vi "recommenceAt.vi"(7 "splitAtFile":path, 10 "Array":path[](array[path])) -> (2 "Array 2":path[](array[path]))   [LabVIEW 2022 SP3]
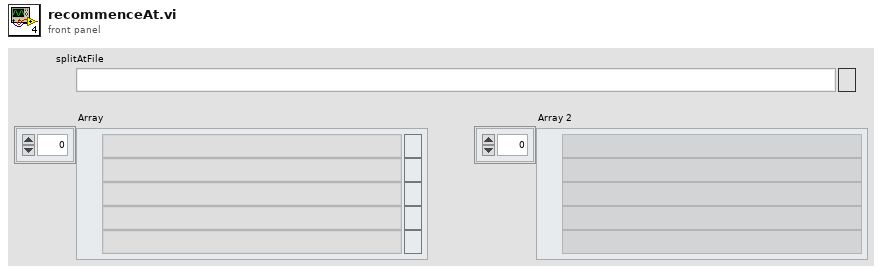
[diagram p1: front panel]
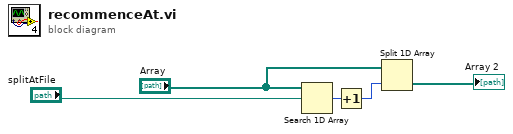
[diagram p0: block diagram]
diagram:
  n1 = Search 1D Array(1D array="Array", element="splitAtFile") -> (index of element=w4:i32)  [unwired: 1 in]
  n2 = Increment(x=w4) -> (x+1=w1:i32)
  n3 = Split 1D Array(array="Array", index=w1) -> (second subarray=→"Array 2":path[])  [unwired: 1 out]
